vi "PQexpressCOPYCmd.vi"(8 "error in (no error)":errorcluster, 10 "Command":string, 11 "conninfo":T1={"host"="localhost", "port"="5432", "client_encoding"="WIN1251", "dbname"="data", "user"="postgres", "password"=""}) -> (0 "error out":errorcluster, 1 "DatabaseMessages":T2, 2 "column_names":string[](array[string]), 3 "data":string[][](array[string]))   [LabVIEW 2019, in "libpqutility.lvlib"]
doc: "use it to get data with COPY function from database\nprovides fast access on plain tables, views and select cmd\n\nPQexpressCmd\nconnect to db\nfire command against db\nget qry result from db\nclose connection\n\nworks only with select cmd \ndoes actually not work with function calls\n\nSee PostgreSQL c-lib doku for further information."
uses:
  libpqutility.lvlib
  libpqlv/src/PQfinish.vi
  libpqlv/src/PQconnectdb.vi
  libpqlv/src/PQerrorMessage.vi
  libpqlv/src/PQstatus.vi
  <vilib>/dlg_ctls.llb/Space Constant.vi
  libpqlv/src/PQnfields.vi
  libpqlv/src/PQgetCopyData.vi
  libpqlv/src/PQfreemem.vi
  libpqlv/src/PQclear.vi
  libpqlv/src/PQcmdTuples.vi
  PQsyncQueryCommand.vi
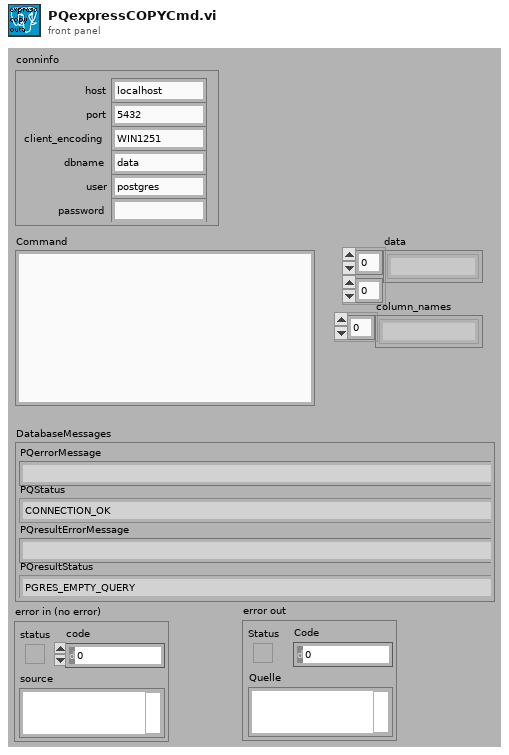
[diagram p1: front panel]
types:
  T1 = cluster{"host":string, "port":string, "client_encoding":string, "dbname":string, "user":string, "password":string}
  T2 = cluster{"PQerrorMessage":string, "PQStatus":enum16{"CONNECTION_OK", "CONNECTION_BAD", "CONNECTION_STARTED", "CONNECTION_MADE", "CONNECTION_AWAITING_RESPONSE", "CONNECTION_AUTH_OK", "CONNECTION_SETENV", "CONNECTION_SSL_STARTUP", "CONNECTION_NEEDED"}, "PQresultErrorMessage":string, "PQresultStatus":enum16{"PGRES_EMPTY_QUERY", "PGRES_COMMAND_OK", "PGRES_TUPLES_OK", "PGRES_COPY_OUT", "PGRES_COPY_IN", "PGRES_BAD_RESPONSE", "PGRES_NONFATAL_ERROR", "PGRES_FATAL_ERROR"}}
  T3 = enum32{"CONNECTION_OK", "CONNECTION_BAD", "CONNECTION_STARTED", "CONNECTION_MADE", "CONNECTION_AWAITING_RESPONSE", "CONNECTION_AUTH_OK", "CONNECTION_SETENV", "CONNECTION_SSL_STARTUP", "CONNECTION_NEEDED"}
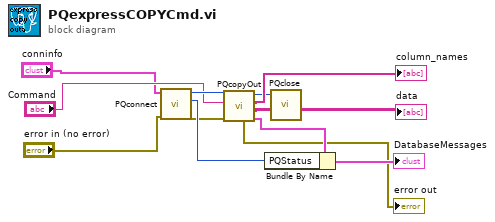
[diagram p0: block diagram]
diagram:
  n1 = call "PQconnect.vi"("error in (no error)"="error in (no error)", "conninfo"="conninfo") -> ("error out"=w1:errorcluster, "PQStatus"=w12:T3, "conn"=w10:u32)  [unwired: 7 in]
  n2 = call "PQcopyOut.vi"("error in (no error)"=w1, "query"="Command", "conn"=w10) -> ("database_status_message"=w8:T2, "data"=→"data":string[][], "column_names"=→"column_names":string[], "conn_out"=w5:u32, "error out"=→"error out":errorcluster)  [unwired: 4 in]
  n3 = Bundle By Name(cluster=w8, "PQStatus"=w12) -> (→"DatabaseMessages":T2)
  n4 = call "PQclose.vi"("conn"=w5) -> ()  [unwired: 10 in, 1 out]
